vi "3D-Cal-4Point-Base.vi"(6 "Labstring":string, 7 "Rectangle":T2 {"Rotation" format="%.2f"; "Left" scale=0.0..1024.0; "Right" scale=0.0..1024.0}, 8 "error in (no error)":errorcluster, 9 "十字线距离":i32, 10 "基准点距离":i32, 11 "Pic Input":T1(plugin-control)) -> (0 "error out":errorcluster, 2 "坐标输出":string[](array[string]), 3 "Pic Output":T1(plugin-control))   [LabVIEW 2015]
panel:
  out "输出簇":cluster{"X":i32, "Y":i32}
  out "Right-a":i32
  out "Bottom+a":i32
  out "Bottom-a":i32
  out "Left+a":i32
  out "Right+a":i32
  out "Top-a":i32
  out "Left-a":i32
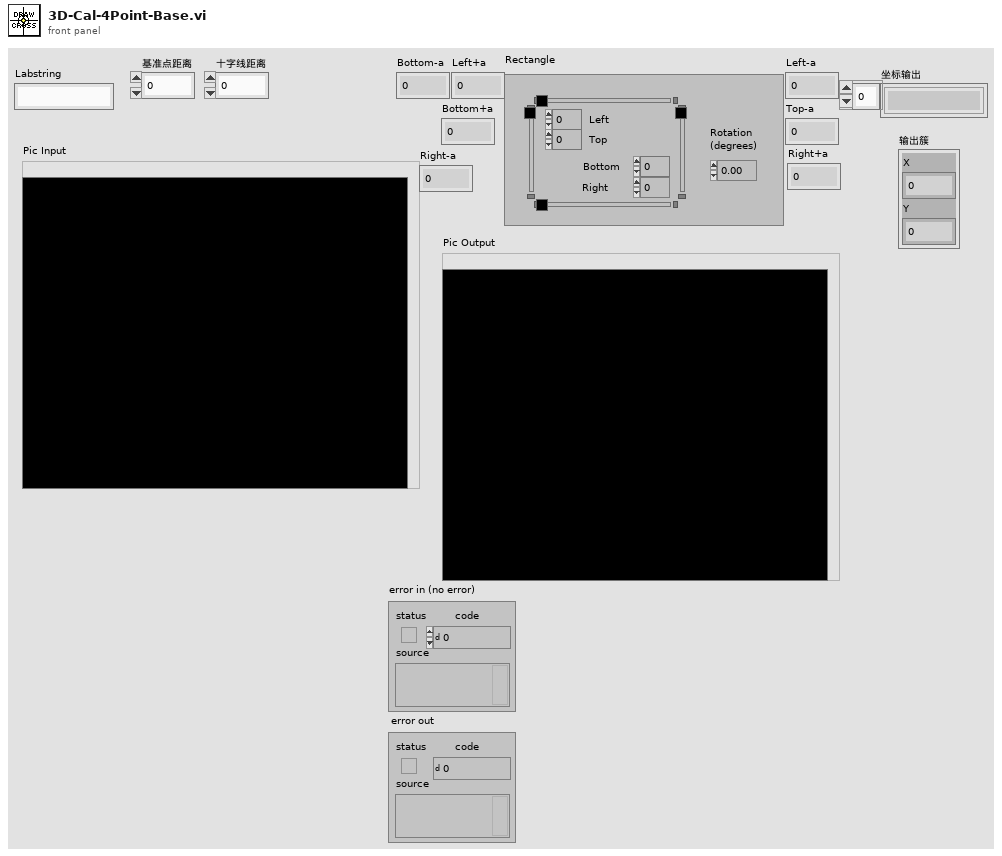
[diagram p1: front panel]
types:
  T1 = typedef "IMAQ Image.ctl" = refnum<image>
  T2 = typedef "IMAQ Rectangle" = cluster{"Left":i32, "Top":i32, "Right":i32, "Bottom":i32, "Rotation":dbl}
  T3 = cluster{"Desired Font (Application)":enum16{"User-specified Font", "Application Font", "System Font", "Dialog Font"}, "[User-specified Font]":cluster{"Font Name":string, "Size":i16, "Strikeout?":bool, "Italic?":bool, "Underline?":bool, "Outline?":bool, "Shadow?":bool, "Bold?":bool, "Rotation Angle":dbl}, "Horizontal Alignment":i16, "Vertical Alignment":i16}
  T4 = cluster{"Left":i32, "Top":i32, "Right":i32, "Bottom":i32}
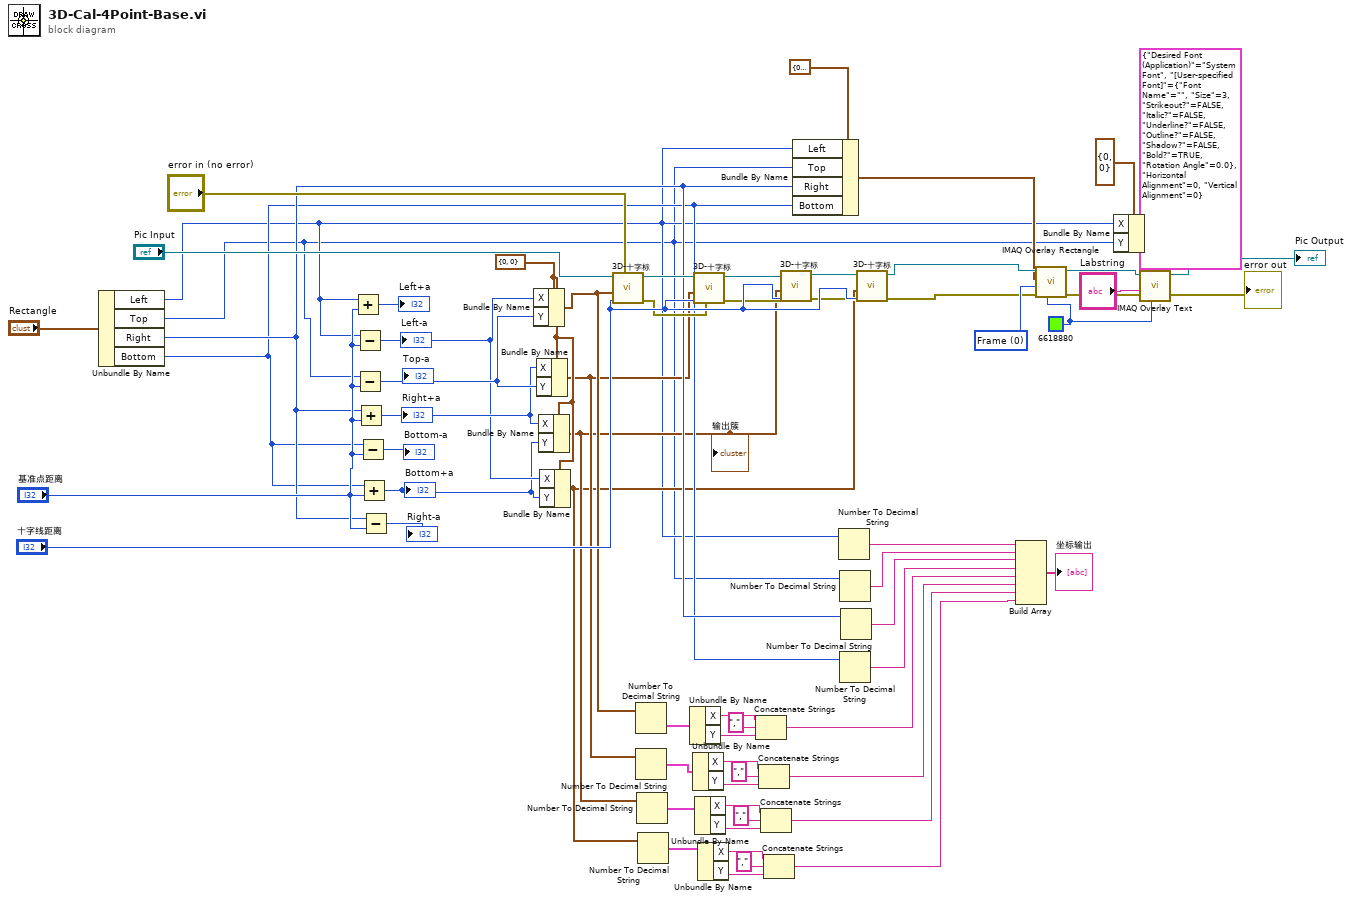
[diagram p0: block diagram]
diagram:
  w54 = u32 0 items=["Frame", "Fill", "Highlight"] ("Drawing Mode (Frame)")
  w1 = u32 6618880
  w63 = cluster{"X":i32, "Y":i32} {"X"=0, "Y"=0} ("CenterPos")
  n1 = Unbundle By Name("Rectangle") -> ("Left"=w4:i32, "Top"=w3:i32, "Right"=w40:i32, "Bottom"=w39:i32)
  n2 = Add(x=w4, y="基准点距离") -> (x+y=→"Left+a":i32)
  n3 = Subtract(x=w4, y="基准点距离") -> (x-y=w43:i32)
  "Left-a" <- w43
  n4 = Subtract(x=w3, y="基准点距离") -> (x-y=w62:i32)
  "Top-a" <- w62
  n5 = Add(x=w40, y="基准点距离") -> (x+y=w44:i32)
  "Right+a" <- w44
  n6 = Subtract(x=w39, y="基准点距离") -> (x-y=→"Bottom-a":i32)
  n7 = Add(x=w39, y="基准点距离") -> (x+y=w41:i32)
  "Bottom+a" <- w41
  n8 = Subtract(x=w40, y="基准点距离") -> (x-y=→"Right-a":i32)
  n9 = Bundle By Name(cluster=w63, "X"=w43, "Y"=w62) -> (w34:cluster{"X":i32, "Y":i32})
  n10 = Bundle By Name(cluster=w63, "X"=w44, "Y"=w62) -> (w33:cluster{"X":i32, "Y":i32})
  n11 = Bundle By Name(cluster=w63, "X"=w44, "Y"=w41) -> (w32:cluster{"X":i32, "Y":i32})
  "输出簇" <- w32
  n12 = Bundle By Name(cluster=w63, "X"=w43, "Y"=w41) -> (w31:cluster{"X":i32, "Y":i32})
  n13 = call "3D-十字标.vi"("error in (no error)"="error in (no error)", "radius"="十字线距离", "CenterPos"=w34, "输入图片"="Pic Input") -> ("error out"=w57:errorcluster, "输出图片"=w64:T1)  [unwired: 6 in]
  n14 = Number To Decimal String(number=w34) -> (decimal integer string=w30:cluster{"X":string, "Y":string})  [unwired: 1 in]
  n15 = Number To Decimal String(number=w33) -> (decimal integer string=w23:cluster{"X":string, "Y":string})  [unwired: 1 in]
  n16 = Number To Decimal String(number=w32) -> (decimal integer string=w19:cluster{"X":string, "Y":string})  [unwired: 1 in]
  n17 = Number To Decimal String(number=w31) -> (decimal integer string=w15:cluster{"X":string, "Y":string})  [unwired: 1 in]
  n18 = Unbundle By Name(w30) -> ("X"=w29:string, "Y"=w27:string)
  n19 = Unbundle By Name(w23) -> ("X"=w24:string, "Y"=w26:string)
  n20 = call "3D-十字标.vi"("error in (no error)"=w57, "radius"="十字线距离", "CenterPos"=w33, "输入图片"=w64) -> ("error out"=w56:errorcluster, "输出图片"=w60:T1)  [unwired: 6 in]
  n21 = Unbundle By Name(w19) -> ("X"=w22:string, "Y"=w20:string)
  n22 = Unbundle By Name(w15) -> ("X"=w16:string, "Y"=w18:string)
  n23 = Concatenate Strings(w29, "," ("X"), w27) -> (w14:string)
  n24 = Concatenate Strings(w24, "," ("X"), w26) -> (w13:string)
  n25 = Concatenate Strings(w22, "," ("X"), w20) -> (w12:string)
  n26 = Concatenate Strings(w16, "," ("X"), w18) -> (w11:string)
  n27 = call "3D-十字标.vi"("error in (no error)"=w56, "radius"="十字线距离", "CenterPos"=w32, "输入图片"=w60) -> ("error out"=w47:errorcluster, "输出图片"=w48:T1)  [unwired: 6 in]
  n28 = Bundle By Name(cluster=T4 {"Left"=0, "Top"=0, "Right"=0, "Bottom"=0} ("Rectangle"), "Left"=w4, "Top"=w3, "Right"=w40, "Bottom"=w39) -> (w51:T4)
  n29 = Number To Decimal String(number=w4) -> (decimal integer string=w38:string)  [unwired: 1 in]
  n30 = Number To Decimal String(number=w3) -> (decimal integer string=w37:string)  [unwired: 1 in]
  n31 = Number To Decimal String(number=w39) -> (decimal integer string=w35:string)  [unwired: 1 in]
  n32 = Number To Decimal String(number=w40) -> (decimal integer string=w36:string)  [unwired: 1 in]
  n33 = call "3D-十字标.vi"("error in (no error)"=w47, "radius"="十字线距离", "CenterPos"=w31, "输入图片"=w48) -> ("error out"=w50:errorcluster, "输出图片"=w55:T1)  [unwired: 6 in]
  n34 = Build Array(w38, w37, w36, w35, w14, w13, w12, w11) -> (→"坐标输出":string[])
  n35 = call "IMAQ Overlay Rectangle"("Color"=w1, "error in (no error)"=w50, "Drawing Mode (Frame)"=w54, "Rectangle"=w51, "Image"=w55) -> ("error out"=→"error out":errorcluster, "Image Out"=w8:T1)  [unwired: 5 in]
  n36 = Bundle By Name(cluster=cluster{"X":i32, "Y":i32} {"X"=0, "Y"=0} ("Origin"), "X"=w4, "Y"=w3) -> (w6:cluster{"X":i32, "Y":i32})
  n37 = call "IMAQ Overlay Text"("Text Color (black)"=w1, "Font, Size & Style"=T3 {"Desired Font (Application)"=enum."System Font", "[User-specified Font]"={"Font Name"="", "Size"=3, "Strikeout?"=FALSE, "Italic?"=FALSE, "Underline?"=FALSE, "Outline?"=FALSE, "Shadow?"=FALSE, "Bold?"=TRUE, "Rotation Angle"=0.0}, "Horizontal Alignment"=0, "Vertical Alignment"=0}, "String"="Labstring", "Origin"=w6, "Image"=w8) -> ("Image Out"=→"Pic Output":T1)  [unwired: 5 in, 1 out]
